vi "Grab First Hit in Boolean Map.vi"(8 "error in (no error)":errorcluster, 11 "Boolean Index Map":refnum<class "2D Array binary.lvclass">) -> (0 "error out":errorcluster, 3 "Backfilled Boolean Index Map":refnum<class "2D Array binary.lvclass">)   [LabVIEW 2020, in "G2CPU Line Profile.lvlib"]
uses:
  G2CPU Line Profile.lvlib
  <vilib>/Natan Biesmans/G2CPU GPU and CPU HPC Toolkit/G2CPU Libraries/Arrays/2DArray/binary/2D Array binary.lvclass
  C:/Program Files/National Instruments/LabVIEW 2025/vi.lib/Natan Biesmans/G2CPU GPU and CPU HPC Toolkit/G2CPU Libraries/Arrays/Array/Array Prototype.lvclass
  <vilib>/Natan Biesmans/G2CPU GPU and CPU HPC Toolkit/G2CPU Libraries/Arrays/Array/Array Prototype.lvclass/Array Prototype.ctl
  8762fac3-58f1-4c7f-909f-b13df01352f1.vi
  528e8d84-4f72-4d39-8363-aa57b5ef4d44.vi
  d68cd2fb-6ccc-4dfd-8692-0ed37b698c6e.vi
  <vilib>/Natan Biesmans/G2CPU GPU and CPU HPC Toolkit/G2CPU Libraries/Arrays/Array/G2CPU Get Array Pointer.vi
  8762fac3-58f1-4c7f-909f-b13df01352f1.vi/e7247370-a01f-465a-ac0e-4dfefcb1bb87.vi
  8762fac3-58f1-4c7f-909f-b13df01352f1.vi/345e91f0-9a5e-4de4-af9c-133346717e4a.vi
  528e8d84-4f72-4d39-8363-aa57b5ef4d44.vi/492a4521-a697-4982-bdb9-a4b473f6765e.vi
  528e8d84-4f72-4d39-8363-aa57b5ef4d44.vi/b6d1f733-f67d-4708-929f-8d6c79a7c52f.vi
  d68cd2fb-6ccc-4dfd-8692-0ed37b698c6e.vi/80f98885-d133-4778-8a71-11569f5a634e.vi
  d68cd2fb-6ccc-4dfd-8692-0ed37b698c6e.vi/fede99c7-5d82-4ae2-b666-3731d213e31f.vi
  528e8d84-4f72-4d39-8363-aa57b5ef4d44.vi/b6d1f733-f67d-4708-929f-8d6c79a7c52f.vi/58bdfdf7-541c-4043-bcec-be03c1e23ff9.vi
  528e8d84-4f72-4d39-8363-aa57b5ef4d44.vi/b6d1f733-f67d-4708-929f-8d6c79a7c52f.vi/7af555d0-5c94-4227-839c-dec32778ebb2.vi
  d68cd2fb-6ccc-4dfd-8692-0ed37b698c6e.vi/80f98885-d133-4778-8a71-11569f5a634e.vi/6058dca8-195d-4566-b47b-6d6a1c5af61f.vi
  d68cd2fb-6ccc-4dfd-8692-0ed37b698c6e.vi/80f98885-d133-4778-8a71-11569f5a634e.vi/6058dca8-195d-4566-b47b-6d6a1c5af61f.vi/77c7badc-ed81-4514-99c1-20d37f4e5ecc.vi
  d68cd2fb-6ccc-4dfd-8692-0ed37b698c6e.vi/80f98885-d133-4778-8a71-11569f5a634e.vi/6058dca8-195d-4566-b47b-6d6a1c5af61f.vi/eb76fa01-6782-47b4-b34f-9eb474c9cc78.vi
  <vilib>/Natan Biesmans/G2CPU GPU and CPU HPC Toolkit/ArrayFire Driver/VIs/Run as Multi Device.vi
  <vilib>/Natan Biesmans/G2CPU GPU and CPU HPC Toolkit/G2CPU Libraries/Arrays/2DArray/s64/2D Array s64.lvclass
  <vilib>/Natan Biesmans/G2CPU GPU and CPU HPC Toolkit/ArrayFire Driver/VIs/cast.vi
  <vilib>/Natan Biesmans/G2CPU GPU and CPU HPC Toolkit/G2CPU Libraries/Arrays/Array/G2CPU Set Array Pointer.vi
  <vilib>/Natan Biesmans/G2CPU GPU and CPU HPC Toolkit/G2CPU Libraries/Arrays/Array/G2CPU Release Array.vi
  <vilib>/Natan Biesmans/G2CPU GPU and CPU HPC Toolkit/ArrayFire Driver/VIs/accum.vi
  <vilib>/Natan Biesmans/G2CPU GPU and CPU HPC Toolkit/G2CPU Libraries/Arrays/SubVI/RemoveReducedDimensionForReorder.vi
  <vilib>/Natan Biesmans/G2CPU GPU and CPU HPC Toolkit/ArrayFire Driver/VIs/reorder.vi
  <vilib>/Natan Biesmans/G2CPU GPU and CPU HPC Toolkit/ArrayFire Driver/VIs/release array.vi
  <vilib>/Natan Biesmans/G2CPU GPU and CPU HPC Toolkit/ArrayFire Driver/VIs/iszero.vi
  <vilib>/Natan Biesmans/G2CPU GPU and CPU HPC Toolkit/ArrayFire Driver/VIs/sub.vi
  <vilib>/Natan Biesmans/G2CPU GPU and CPU HPC Toolkit/ArrayFire Driver/subvi/Error Converter (ErrCode or Status).vi
  <vilib>/Natan Biesmans/G2CPU GPU and CPU HPC Toolkit/ArrayFire Driver/VIs/add.vi
  <vilib>/Natan Biesmans/G2CPU GPU and CPU HPC Toolkit/ArrayFire Driver/VIs/ge.vi
  <vilib>/Natan Biesmans/G2CPU GPU and CPU HPC Toolkit/G2CPU Libraries/Arrays/Array/Array Prototype.lvclass
  <vilib>/Natan Biesmans/G2CPU GPU and CPU HPC Toolkit/G2CPU Libraries/Arrays/2DArray/2D Array Prototype.lvclass
  <vilib>/Natan Biesmans/G2CPU GPU and CPU HPC Toolkit/G2CPU Libraries/Arrays/DataTypes/I64/s64.lvclass
  <vilib>/Natan Biesmans/G2CPU GPU and CPU HPC Toolkit/G2CPU Libraries/Arrays/1DArray/s64/1D Array s64.lvclass
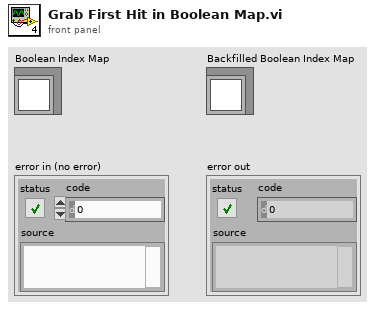
[diagram p1: front panel]
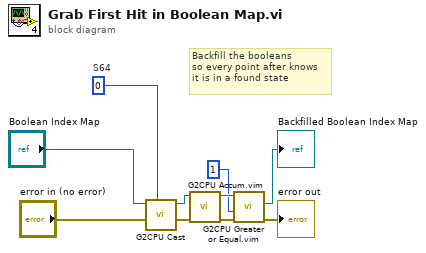
[diagram p0: block diagram]
diagram:
  w10 = i64 0  # S64
  # "Backfill the booleans\nso every point after knows\nit is in a found state"
  n1 = call "G2CPU Cast"("Datatype Prototype"=w10, "error in (no error)"="error in (no error)", "Array In"="Boolean Index Map") -> ("error out"=w7:errorcluster, "Array Out"=w2:refnum<class "2D Array s64.lvclass">)  [unwired: 7 in]
  n2 = call "G2CPU Accum.vim"("error in (no error)"=w7, "Array in"=w2) -> ("error out"=w6:errorcluster, "Array Result"=w5:refnum<class "2D Array s64.lvclass">)  [unwired: 8 in]
  n3 = call "G2CPU Greater or Equal.vim"("error in (no error)"=w6, "Array rhs"=i64 1 ("Datatype Prototype"), "Array lhs"=w5) -> ("error out"=→"error out":errorcluster, "Array Result"=→"Backfilled Boolean Index Map":refnum<class "2D Array binary.lvclass">)  [unwired: 7 in]
